vi "Get Value.vi"(8 "error in (no error)":errorcluster, 11 "Timestamp Item Configuration in":refnum<class "Timestamp Item Configuration.lvclass">) -> (0 "error out":errorcluster, 2 "Project Info Value":string, 3 "Timestamp Item Configuration out":refnum<class "Timestamp Item Configuration.lvclass">)   [LabVIEW 2013, in "Item Configuration.lvlib" / "Timestamp Item Configuration.lvclass"]
uses:
  Timestamp Item Configuration.lvclass
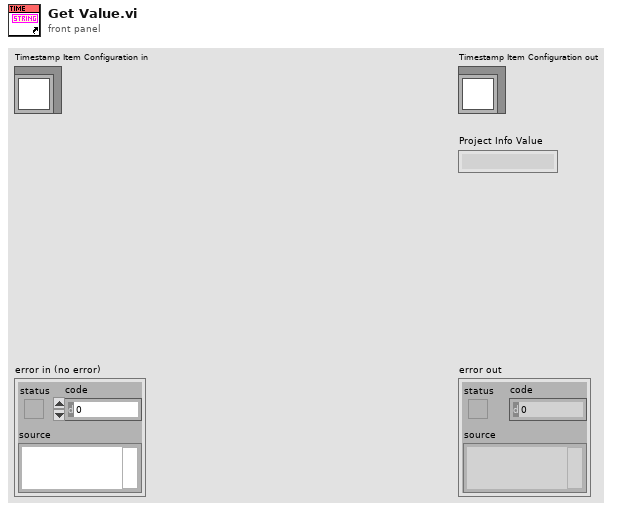
[diagram p1: front panel]
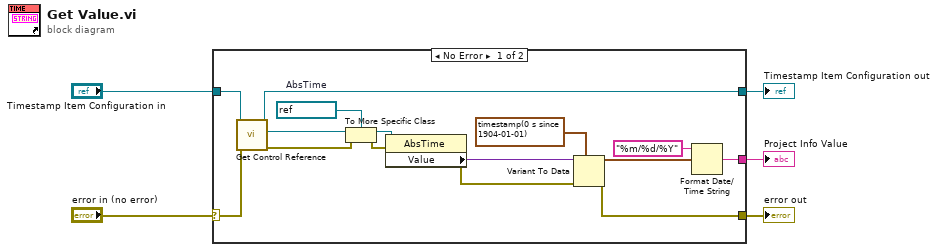
[diagram p0: block diagram]
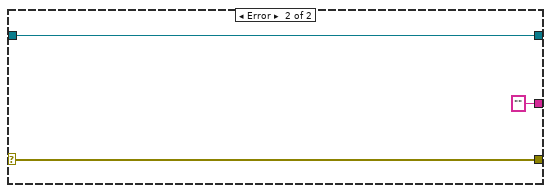
[diagram p2: hidden frame]
diagram:
  n1 = case shown="No Error" "error in (no error)" {
    selector: "error in (no error)" -> [w8 w23]
    tunnel: "Timestamp Item Configuration in" -> [w20 w21]
    tunnel: [w9 "" ("date/time string")] -> w4
    tunnel: [w6 w23] -> w2
    tunnel: [w7 w21] -> w1
    frame No Error {
      w18 = refnum<vi> refnum  # AbsTime
      n2 = call-dynamic "Get Control Reference.vi"("error in (no error)"=w8, "Item Configuration in"=w20) -> ("error out"=w17:errorcluster, "Control Reference"=w19:refnum<vi>, "Item Configuration out"=w7:refnum<class "Timestamp Item Configuration.lvclass">)  [unwired: 7 in]
      n3 = To More Specific Class(target class=w18, reference=w19, error in=w17) -> (specific class reference=w15:refnum<vi>, error out=w16:errorcluster)
      n4 = property class="AbsTime"(reference=w15, error in=w16) -> (error out=w10:errorcluster, "Value"=w14:variant)  [unwired: 1 out]
      n5 = Variant To Data(error in=w10, type=timestamp(0 s since 1904-01-01) ("current time"), Variant=w14) -> (data=w12:timestamp, error out=w6:errorcluster)
      n6 = Format Date/Time String(time format string (%c)="%m/%d/%Y", seconds (now)=w12) -> (date/time string=w9:string)  [unwired: 1 in]
    }
    frame Error {
    }
  }
  "error out" <- w2
  "Timestamp Item Configuration out" <- w1
  "Project Info Value" <- w4
